vi "fpga_Reset State.vi"(8 "input valid":bool=TRUE, 11 "channel index":u8) -> (3 "reset?":bool)   [LabVIEW 2012, in "NI_EP_Protection_FPGA.lvlib"]
uses:
  <vilib>/addons/Electrical Power/Protection/NI_EP_Protection_FPGA.lvlib
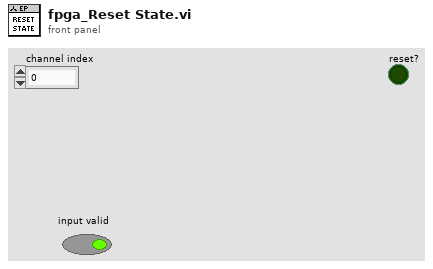
[diagram p1: front panel]
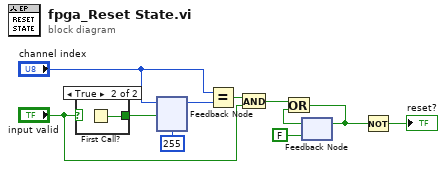
[diagram p0: block diagram]
diagram:
  n1 = case shown="True" "input valid" {
    tunnel: [_ w12] -> w4
    frame False {
    }
    frame True {
      n2 = First Call?() -> (First Call?: T/F=w12:bool)
    }
  }
  n3 = feedback #1(u8 255 ("channel index")) -> (w10:u8)
  n4 = feedback-in #1("channel index", w4) -> ()
  n5 = Equal?(x="channel index", y=w10) -> (x = y?=w9:bool)
  n6 = And(x=w9, y="input valid") -> (x .and. y?=w6:bool)
  n7 = feedback #2(FALSE) -> (w8:bool)
  n8 = Or(x=w6, y=w8) -> (x .or. y?=w5:bool)
  n9 = feedback-in #2(w5) -> ()
  n10 = Not(x=w5) -> (.not. x?=→"reset?":bool)
